vi "Matrix_Multiply_v1.vi"() -> ()   [LabVIEW 2020]
uses:
  <vilib>/Analysis/Matrix/Datatypes/RealMatrix.ctl
  <vilib>/Analysis/baseanly.llb/Real A x B.vi
  <vilib>/Analysis/Matrix/Numeric/Conversions/Matrix To Array - RM.vi
  <vilib>/Analysis/NI_AALBase.lvlib
  <vilib>/Analysis/Matrix/NI_Matrix.lvlib
panel:
  in  "num of col for B (p)":i32=1
  in  "num of col for A (n)":i32=7
  in  "num of rows (m)":i32=3
  out "sum of error":dbl
  out "Array 3":i32[](array[numeric])
  out "Array 2":i32[][](array[numeric])
  out "output array":sgl[][](array[numeric])
  out "Array":dbl[](array[numeric])
  out "1D array of C":sgl[](array[numeric])
  out "a":i32[](array[numeric])
  out "b":i32[](array[numeric])
  out "A x B":T1
  out "Numeric":dbl
  out "n":i32=10
  out "m":i32=10
  out "p":i32=10
  out "Real 2D Array":dbl[][](array[numeric])
  out "B":dbl[][](array[numeric])
  out "1D array of A":dbl[](array[numeric])
  out "A":dbl[][](array[numeric])
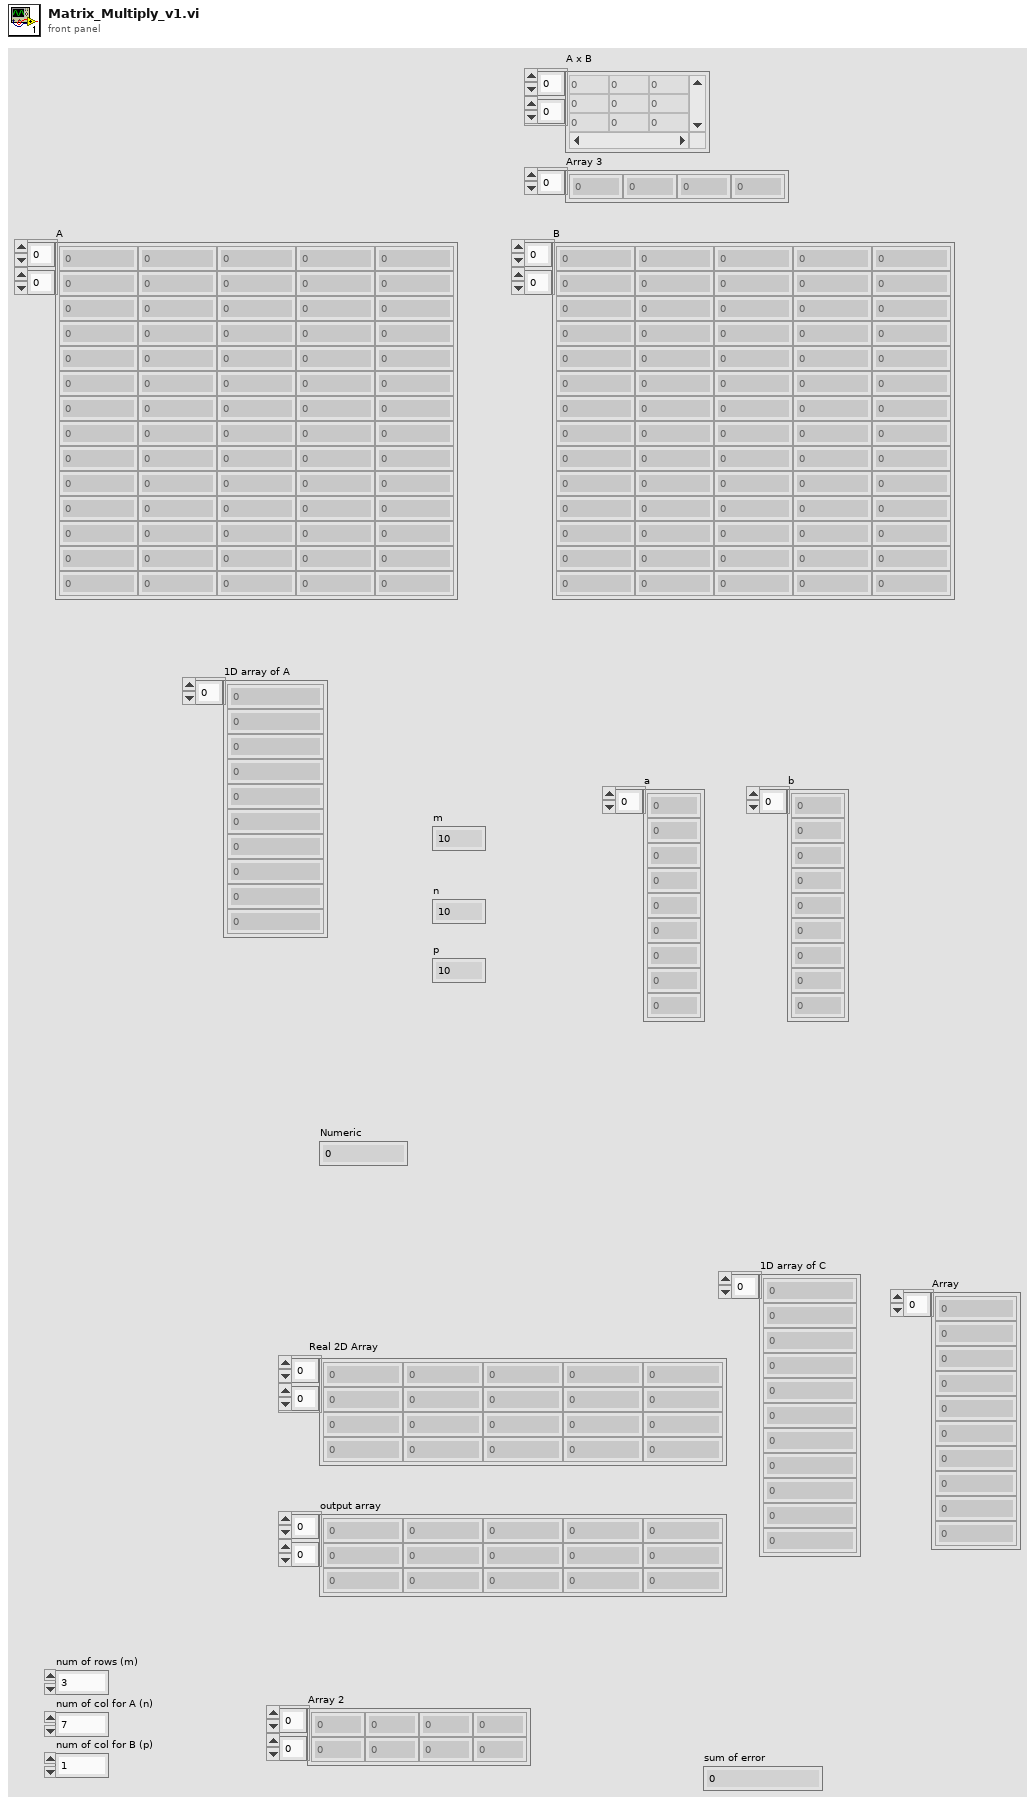
[diagram p1: front panel]
types:
  T1 = typedef "NI_Matrix.lvlib/RealMatrix.ctl" = dbl[][]
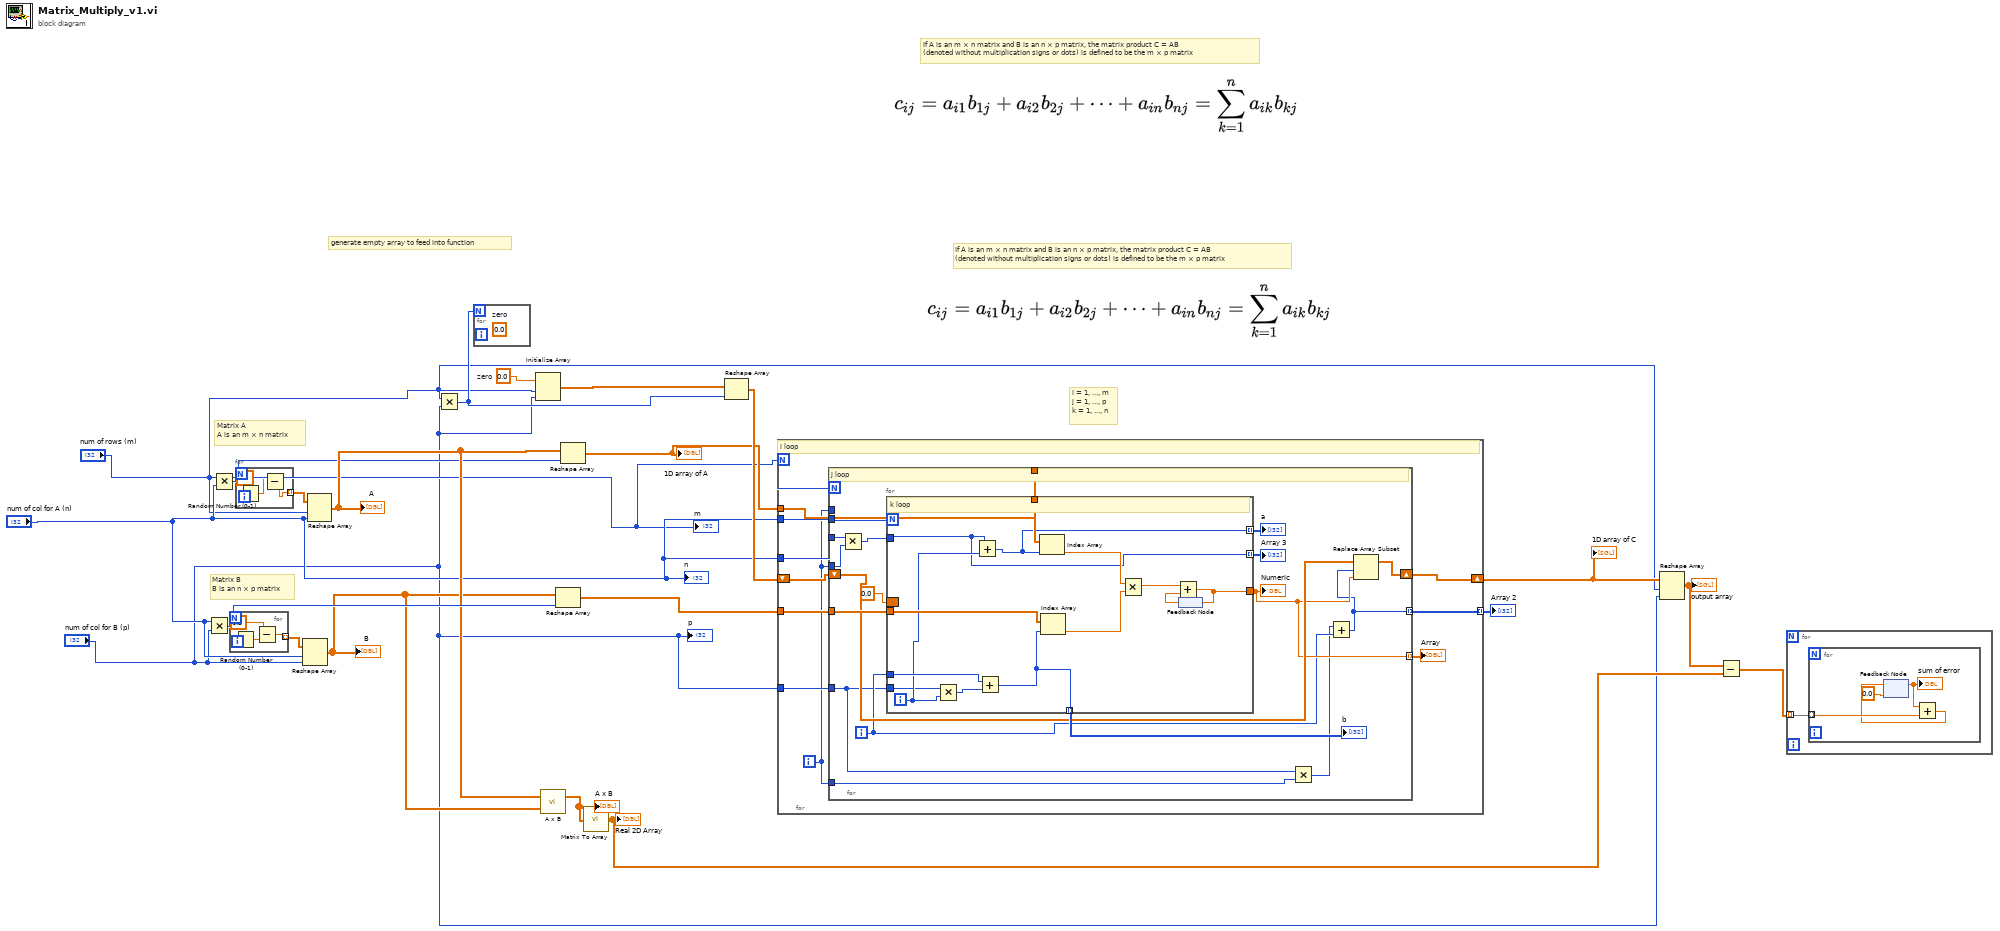
[diagram p0: block diagram]
diagram:
  w18 = sgl 0.0  # zero
  # "If A is an m × n matrix and B is an n × p matrix, the matrix product C = AB \n(denoted without multiplication signs or dots) is defined to be the m × p matrix"
  # "If A is an m × n matrix and B is an n × p matrix, the matrix product C = AB \n(denoted without multiplication signs or dots) is defined to be the m × p matrix"
  # "i = 1, ..., m\nj = 1, ..., p\nk = 1, ..., n"
  # "generate empty array to feed into function"
  # "Matrix B\nB is an n × p matrix"
  # "Matrix A\nA is an m × n matrix"
  n1 = Multiply(x="num of col for A (n)", y="num of col for B (p)") -> (x*y=w19:i32)
  n2 = Multiply(x="num of rows (m)", y="num of col for A (n)") -> (x*y=w13:i32)
  n3 = for {
    N: w19 -> [_]
    tunnel: [w23] -> w20 mode=indexing
    n4 = Random Number (0-1)() -> (number: 0 to 1=w24:dbl)
    n5 = Subtract(x=w24, y=0.5) -> (x-y=w23:dbl)
  }
  n6 = for {
    N: w13 -> [_]
    tunnel: [w26] -> w21 mode=indexing
    n7 = Random Number (0-1)() -> (number: 0 to 1=w27:dbl)
    n8 = Subtract(x=w27, y=0.5) -> (x-y=w26:dbl)
  }
  n9 = Reshape Array(w20, "num of col for A (n)", "num of col for B (p)") -> (w16:dbl[][])
  "B" <- w16
  n10 = Reshape Array(w21, "num of rows (m)", "num of col for A (n)") -> (w17:dbl[][])
  "A" <- w17
  n11 = Multiply(x="num of rows (m)", y="num of col for B (p)") -> (x*y=w10:i32)
  n12 = for {
    N: w10 -> [_]
    (unwired) sgl 0.0  # zero
  }
  n13 = Initialize Array(w18, "num of rows (m)", "num of col for B (p)") -> (w14:sgl[][])
  n14 = call-poly <vilib>:"A x B.vi"("B"=w16, "A"=w17) -> ("A x B"=w15:T1)  [unwired: 1 out]
  "A x B" <- w15
  n15 = Reshape Array(w16, w19) -> (w12:dbl[])
  n16 = Reshape Array(w17, w13) -> (w8:dbl[])
  "1D array of A" <- w8
  n17 = call-poly <vilib>:"Matrix To Array.vi"("Real Matrix"=w15) -> ("Real 2D Array"=w5:dbl[][])
  "Real 2D Array" <- w5
  n18 = Reshape Array(w14, w10) -> (w11:sgl[])
  n19 = for {
    N: "num of rows (m)" -> [_]
    tunnel: w12 -> [w37]
    tunnel: "num of col for A (n)" -> [w36]
    tunnel: "num of col for B (p)" -> [w32]
    tunnel: w8 -> [w31]
    tunnel: [w30] -> w7 mode=indexing
    tunnel: "num of col for A (n)" -> [w29]
    shift-right: [w33] -> w9
    shift-left: w11 -> [w35]
    i -> [w28]
    # "i loop"
    n20 = for {
      N: w32 -> [_]
      tunnel: w31 -> [w55]
      tunnel: w28 -> [_]
      tunnel: w37 -> [w54]
      tunnel: w36 -> [w46]
      tunnel: w32 -> [w38]
      tunnel: [w48] -> w34 mode=indexing
      tunnel: [w47] -> w30 mode=indexing
      shift-right: [w49] -> w33
      shift-left: w35 -> [w50]
      tunnel: w28 -> [w44]
      tunnel: w29 -> [w42]
      tunnel: w28 -> [w40]
      i -> [w45]
      # "j loop"
      n21 = Multiply(x=w42, y=w40) -> (x*y=w41:i32)
      n22 = for {
        N: w46 -> [_]
        tunnel: w55 -> [w69]
        tunnel: w41 -> [w56]
        tunnel: w54 -> [w68]
        tunnel: w45 -> [w62]
        tunnel: [w63] -> w48
        tunnel: w38 -> [w60]
        tunnel: [w58] -> w53 mode=indexing
        tunnel: [w57] -> w52 mode=indexing
        border: 0.0 -> [_]
        tunnel: [w56] -> w39 mode=indexing
        i -> [w61]
        # "k loop"
        n23 = Multiply(x=w60, y=w61) -> (x*y=w59:i32)
        n24 = Add(x=w56, y=w61) -> (x+y=w57:i32)
        n25 = Add(x=w62, y=w59) -> (x+y=w58:i32)
        n26 = Index Array(array=w69, index=w57) -> (element=w67:dbl)
        n27 = Index Array(array=w68, index=w58) -> (element=w66:dbl)
        n28 = Multiply(x=w67, y=w66) -> (x*y=w65:dbl)
        n29 = feedback #1() -> (w64:dbl)
        n30 = Add(x=w65, y=w64) -> (x+y=w63:dbl)
        n31 = feedback-in #1(w63) -> ()
      }
      "Numeric" <- w48
      "b" <- w53
      "a" <- w52
      "Array 3" <- w39
      n32 = Multiply(x=w38, y=w44) -> (x*y=w43:i32)
      n33 = Add(x=w43, y=w45) -> (x+y=w47:i32)
      n34 = Replace Array Subset(array=w50, new element=w48, index=w47) -> (w49:sgl[])
    }
    "Array" <- w34
  }
  "1D array of C" <- w9
  "Array 2" <- w7
  n35 = Reshape Array(w9, "num of rows (m)", "num of col for B (p)") -> (w6:sgl[][])
  "output array" <- w6
  n36 = Subtract(x=w6, y=w5) -> (x-y=w4:dbl[][])
  n37 = for {
    tunnel: w4 -> [w70] mode=indexing
    n38 = for {
      tunnel: w70 -> [w74] mode=indexing
      n39 = feedback #2(0.0) -> (w72:dbl)
      "sum of error" <- w72
      n40 = Add(x=w72, y=w74) -> (x+y=w73:dbl)
      n41 = feedback-in #2(w73) -> ()
    }
  }
  "p" <- "num of col for B (p)"
  "m" <- "num of rows (m)"
  "n" <- "num of col for A (n)"
